vi "VISA_test.vi"() -> ()   [LabVIEW 2016]
uses:
  <vilib>/Instr/_visa.llb/VISA Configure Serial Port (Instr).vi
panel:
  out "2 Channel signal":cluster{u8, u8}(graph)
  in  "Channel 2":dbl=1.0
  in  "Channel":dbl=6.0
  out "Value":u8
  out "8 Channel value":u8[](array[numeric])
  out "Signal":u8(graph)
  in  "stop bits (10: 1 bit)":u16(ring)=10 items=["1.0"=10, "1.5"=15, "2.0"=20]
  in  "termination char\n(0xA = '\\n' = LF)":u8=53 format="%.0x"
  in  "data bits (8)":u16=8 min=5 max=8 step=1
  in  "baud rate (115200)":u32=115200
  out "read buffer":string
  in  "VISA resource name":refnum<visa-resource-name>="COM3"
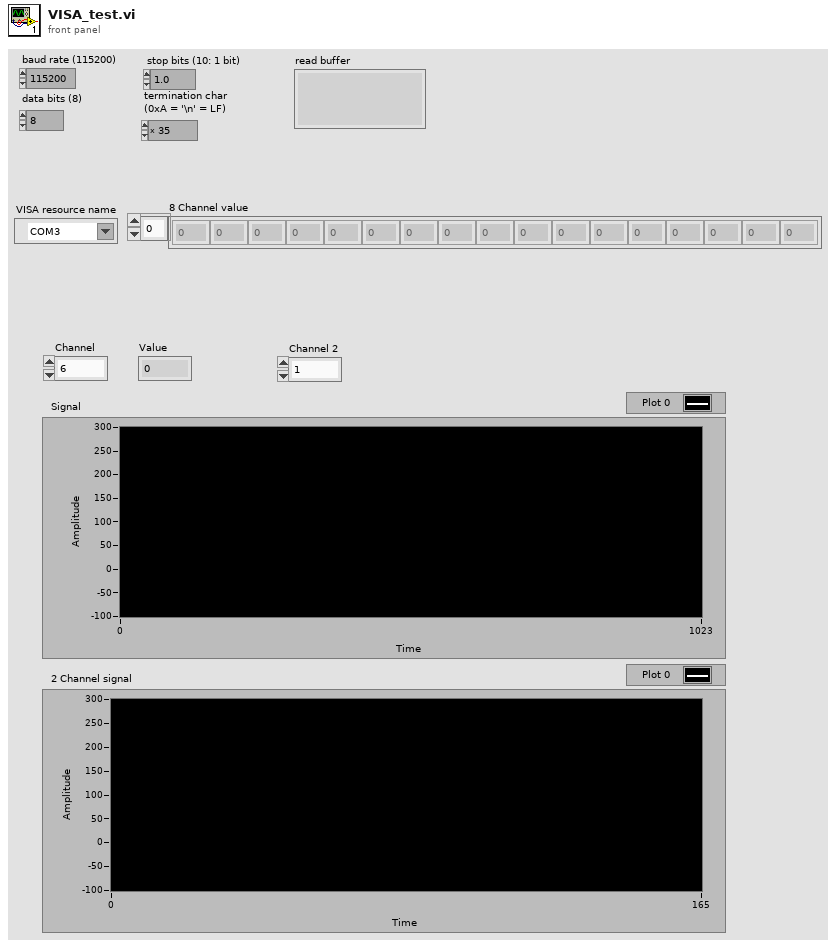
[diagram p1: front panel]
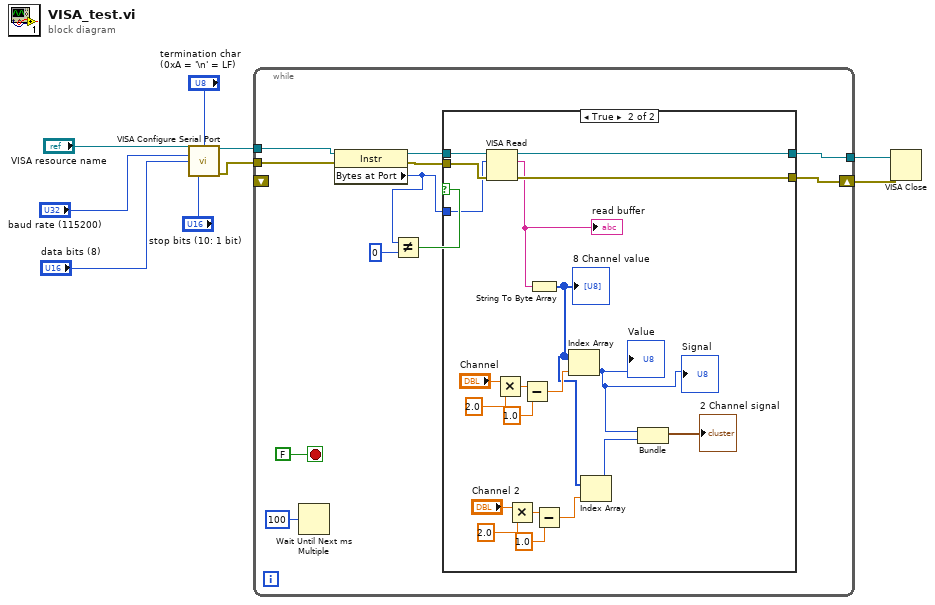
[diagram p0: block diagram]
diagram:
  n1 = call-poly "VISA Configure Serial Port"("VISA resource name"="VISA resource name", "termination char\n(0xA = '\\n' = LF)"="termination char\n(0xA = '\\n' = LF)", "baud rate (115200)"="baud rate (115200)", "data bits (8)"="data bits (8)", "stop bits (10: 1 bit)"="stop bits (10: 1 bit)") -> ("VISA resource name out"=w2:refnum<visa-resource-name>, "error out"=w1:errorcluster)  [unwired: 9 in]
  n2 = while {
    shift-right: [w19] -> w3
    shift-left: _ -> [_]
    tunnel: [w20] -> w4
    tunnel: w2 -> [w17]
    tunnel: w1 -> [w15]
    stop <- FALSE stop-if-true
    n3 = Wait Until Next ms Multiple(millisecond multiple=u32 100) -> ()  [unwired: 1 out]
    n4 = property class="Instr"(reference=w17, error in=w15) -> (reference out=w16:refnum<visa-resource-name>, error out=w14:errorcluster, "Bytes at Port"=w13:u32)
    n5 = Not Equal?(x=w13, y=u32 0) -> (x != y?=w11:bool)
    n6 = case shown="True" w11 {
      tunnel: [w22 w42] -> w20
      tunnel: [w21 w41] -> w19
      tunnel: w16 -> [w22 w40]
      tunnel: w14 -> [w21 w39]
      tunnel: w13 -> [_ w38]
      frame False {
      }
      frame True {
        n7 = VISA Read(VISA resource name=w40, byte count=w38, error in (no error)=w39) -> (VISA resource name out=w42:refnum<visa-resource-name>, read buffer=w37:string, error out=w41:errorcluster)  [unwired: 1 out]
        "read buffer" <- w37
        n8 = Multiply(x="Channel", y=2.0) -> (x*y=w32:dbl)
        n9 = Multiply(x="Channel 2", y=2.0) -> (x*y=w27:dbl)
        n10 = Subtract(x=w32, y=1.0) -> (x-y=w33:dbl)
        n11 = String To Byte Array(string=w37) -> (unsigned byte array=w26:u8[])
        "8 Channel value" <- w26
        n12 = Subtract(x=w27, y=1.0) -> (x-y=w28:dbl)
        n13 = Index Array(array=w26, index=w33) -> (element=w25:u8)
        "Signal" <- w25
        "Value" <- w25
        n14 = Index Array(array=w26, index=w28) -> (element=w24:u8)
        n15 = Bundle(w25, w24) -> (→"2 Channel signal":cluster{u8, u8})  [unwired: 1 in]
      }
    }
  }
  n16 = VISA Close(VISA resource name=w4, error in (no error)=w3) -> ()  [unwired: 1 out]
